vi "ManualCommands.vi"(1 "Command to send":string) -> (0 "Reply received":string="***")   [LabVIEW 2014]
panel:
  out "Error":bool
  in  "Send":bool
  in  "Exit":bool
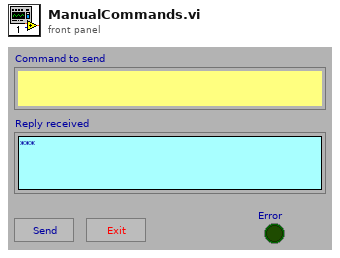
[diagram p1: front panel]
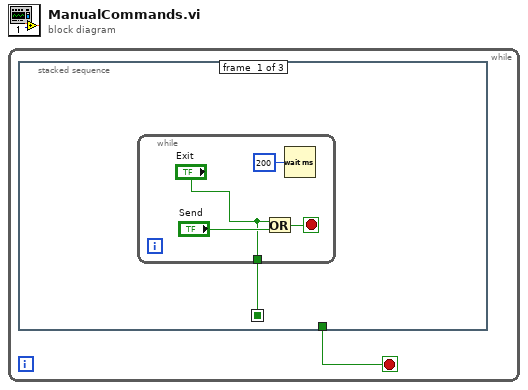
[diagram p0: block diagram]
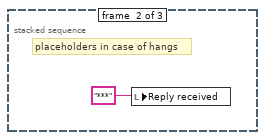
[diagram p2: hidden frame]
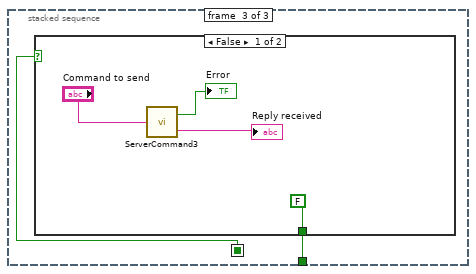
[diagram p3: hidden frame]
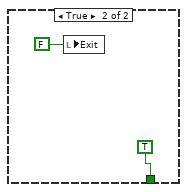
[diagram p4: hidden frame]
diagram:
  n1 = while {
    stop <- w1 stop-if-true
    n2 = stacked-sequence {
      seq-local: [w2 _ _] -> [_ _ w8]
      tunnel: [_ _ w9] -> w1
      frame #0 {
        n3 = while {
          tunnel: ["Exit"] -> w2
          stop <- w5 stop-if-true
          n4 = Or(x="Exit", y="Send") -> (x .or. y?=w5:bool)
          n5 = Wait (ms)(milliseconds to wait=u32 200) -> ()  [unwired: 1 out]
        }
      }
      frame #1 {
        # "placeholders in case of hangs"
        n6 = local write "Reply received"("***" ("reply received")) -> ()
      }
      frame #2 {
        n7 = case shown="False" w8 {
          tunnel: [FALSE TRUE] -> w9
          frame False {
            n8 = call "ServerCommand3.vi"("Command"="Command to send") -> ("Error"=→"Error":bool, "Reply"=→"Reply received":string)
          }
          frame True {
            n9 = local write "Exit"(FALSE ("stop")) -> ()
          }
        }
      }
    }
  }
